vi "Set AccessType.vi"(8 "error in (no error)":errorcluster, 10 "AccessType":T1={"AccessType"=enum."Ro", "Null"=TRUE}, 11 "PDO Communication Parameter in":refnum<class "PDO Communication Parameter.lvclass">) -> (0 "error out":errorcluster, 3 "PDO Communication Parameter out":refnum<class "PDO Communication Parameter.lvclass">)   [LabVIEW 2019, in "PDO Grid.lvlib" / "PDO Communication Parameter.lvclass"]
uses:
  PDO Communication Parameter.lvclass
  PDO Communication Parameter.lvclass/PDO Communication Parameter.ctl
  Access Type.ctl
  Electronic Datasheet.lvlib
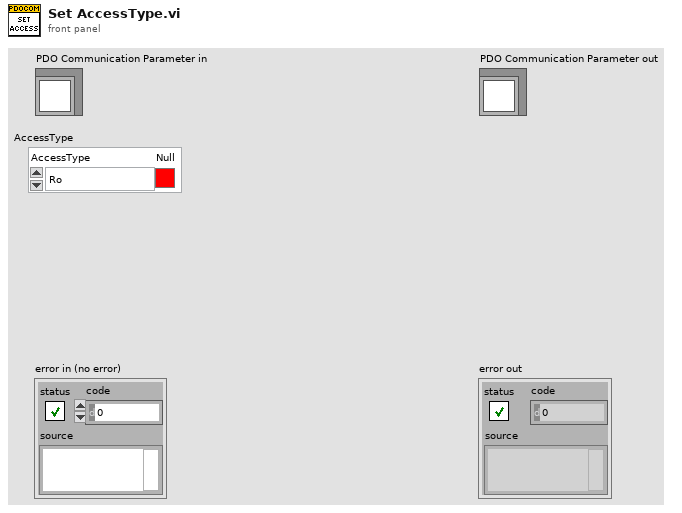
[diagram p1: front panel]
types:
  T1 = typedef "Electronic Datasheet.lvlib/Access Type.ctl" = cluster{"AccessType":enum16{"Ro", "Wo", "Rw", "Const", "Unknown"}, "Null":bool}
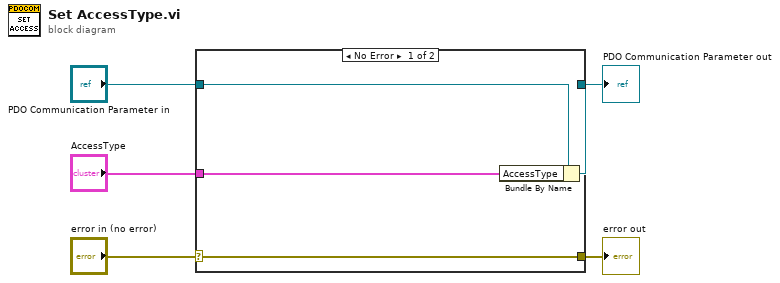
[diagram p0: block diagram]
diagram:
  n1 = case shown="No Error" "error in (no error)" {
    selector: "error in (no error)" -> [w9 w10]
    tunnel: [w9 w10] -> w4
    tunnel: [w7 w11] -> w2
    tunnel: "PDO Communication Parameter in" -> [w8 w11]
    tunnel: "AccessType" -> [w6 _]
    frame No Error {
      n2 = Bundle By Name(cluster=w8, "AccessType"=w6) -> (w7:refnum<class "PDO Communication Parameter.lvclass">)
    }
    frame Error {
    }
  }
  "error out" <- w4
  "PDO Communication Parameter out" <- w2
